vi "Read Power.vi"(0 "SG Path Power Meter Accessor in":refnum<class "SG Path Accessor.lvclass">, 5 "Cal point in":T1, 11 "error in":errorcluster) -> (4 "SG Path Power Meter Accessor out":refnum<class "SG Path Accessor.lvclass">, 6 "Power (dBm)":dbl, 15 "error out":errorcluster)   [LabVIEW 2023, in "NI Cal-5501 Power Detector.lvlib" / "SG Path Accessor.lvclass"]
uses:
  SG Path Accessor.lvclass
  Public/Base Classes/Scalar/Scalar Path/Type Definitions/Cal Point.ctl
  Power Detector/Power Detector.lvclass
  Power Detector/Power Detector.lvclass/Power Detector.ctl
  Power Detector/Properties/Read Resource Name.vi
  Instruments/Power Meter/Power Meter Factory/Power Meter Factory.lvclass
  Public/Base Classes/Scalar/Scalar Path/Scalar Path.lvclass
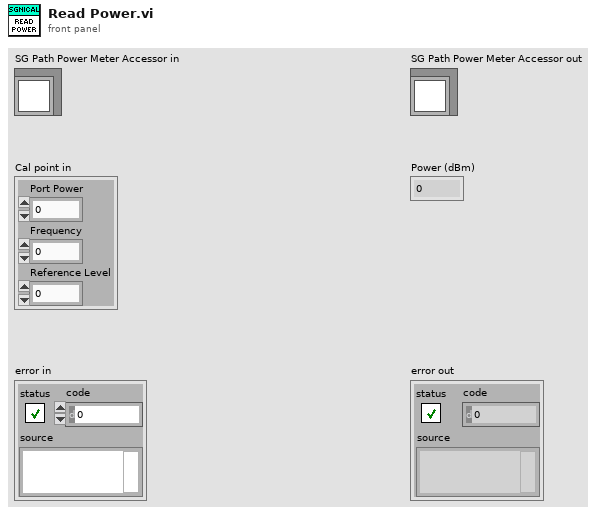
[diagram p1: front panel]
types:
  T1 = typedef "RFFixtureCharact.Public.lvlib/Scalar Path.lvclass/Cal Point.ctl" = cluster{"Port Power":dbl, "Frequency":dbl, "Reference Level":dbl}
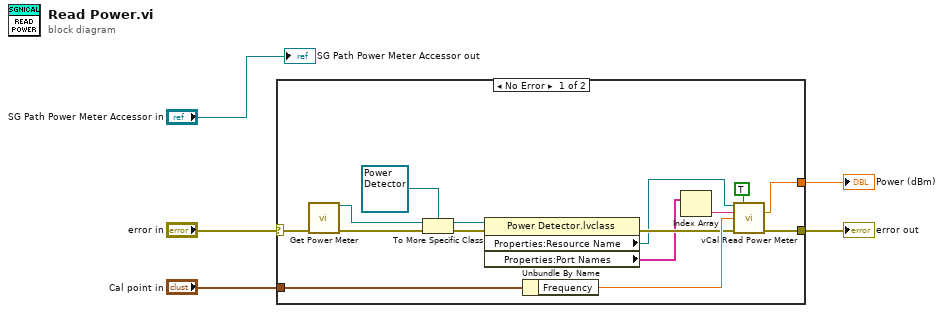
[diagram p0: block diagram]
diagram:
  n1 = case shown="No Error" "error in" {
    selector: "error in" -> [w20 w21]
    tunnel: [w13 w21] -> w4
    tunnel: [w15 _] -> w5
    tunnel: "Cal point in" -> [w11 _]
    frame No Error {
      n2 = call "Get Power Meter.vi"("error in (no error)"=w20) -> ("Power Meter Base out"=w17:refnum<class "Power Meter Base.lvclass">, "error out"=w16:errorcluster)  [unwired: 13 in]
      n3 = To More Specific Class(target class=refnum<class "Power Detector.lvclass"> refnum ("Power Detector"), reference=w17, error in=w16) -> (specific class reference=w18:refnum<class "Power Detector.lvclass">, error out=w19:errorcluster)
      n4 = property class="Power Detector.lvclass"(reference=w18, error in=w19) -> (error out=w9:errorcluster, "Properties:Resource Name"=w6:refnum<k15>, "Properties:Port Names"=w7:string[])  [unwired: 1 out]
      n5 = Unbundle By Name(w11) -> ("Frequency"=w10:dbl)
      n6 = Index Array(array=w7) -> (element=w8:string)  [unwired: 1 in]
      n7 = call <instrlib>:"vCal Read Power Meter.vi"("instrument handle"=w6, "apply temperature compensation"=TRUE, "port name"=w8, "frequency"=w10, "error in"=w9) -> ("power meter value"=w15:dbl, "error out"=w13:errorcluster)  [unwired: 8 in, 1 out]
    }
    frame Error {
    }
  }
  "error out" <- w4
  "Power (dBm)" <- w5
  "SG Path Power Meter Accessor out" <- "SG Path Power Meter Accessor in"
